vi "Monitors_v01.vi"() -> ()   [LabVIEW 2013]
uses:
  <vilib>/Analysis/5stat.llb/RMS (DBL).vi
  <vilib>/Analysis/baseanly.llb/Mean (DBL).vi
  <vilib>/measure/macond.llb/IIR Filter for N Chan.vi
  Global VIs/shotnoise.vi
  <vilib>/Analysis/NI_AALPro.lvlib
  <vilib>/Analysis/NI_AALBase.lvlib
  <vilib>/measure/NI_MAPro.lvlib
panel:
  in  "IIR filter specifications":T1={"Topology"=enum."Butterworth", "Type"=enum."Lowpass", "Order"=1, "Lower Fc"=100.0, "Upper Fc"=200.0, "PB Ripple"=1.0, "SB Attenuation"=60.0} {"PB Ripple" format="%0.2f"; "SB Attenuation" format="%0.2f"; "Lower Fc" format="%0.2p"; "Upper Fc" format="%0.2p"}
  in  "Shot noise start":bool
  out "Variance 1 normalised to SNL":dbl(graph)
  out "Variance 2 normalised to SNL":dbl(graph)
  out "conditional variance":dbl
  out "covariance":dbl
  out "Signal 2":dbl[](graph)
  out "Signal 1":dbl[](graph)
  in  "wfm":waveform(dbl)[](array[waveform]) caption="波形"
types:
  T1 = cluster{"Topology":enum16{"Off", "Butterworth", "Chebyshev", "Inverse Chebyshev", "Elliptic", "Bessel"}, "Type":enum16{"Lowpass", "Highpass", "Bandpass", "Bandstop"}, "Order":i32, "Lower Fc":dbl, "Upper Fc":dbl, "PB Ripple":dbl, "SB Attenuation":dbl}
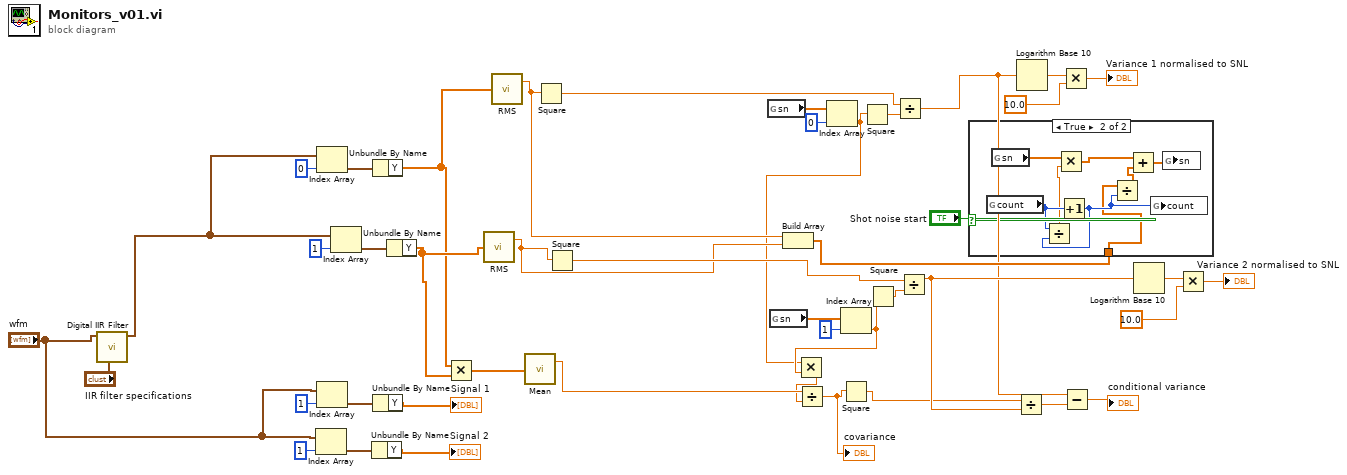
[diagram p0: block diagram]
diagram:
  n1 = call-poly <vilib>:"Digital IIR Filter.vi"("IIR filter specifications"="IIR filter specifications", "signal(s) in"="wfm") -> ("signal(s) out"=w1:waveform(dbl)[])  [unwired: 4 in, 5 out]
  n2 = Index Array(array="wfm", index=1) -> (element=w40:waveform(dbl))
  n3 = Index Array(array=w1, index=0) -> (element=w12:waveform(dbl))
  n4 = Index Array(array="wfm", index=1) -> (element=w43:waveform(dbl))
  n5 = Index Array(array=w1, index=1) -> (element=w17:waveform(dbl))
  n6 = Unbundle By Name(w40) -> ("Y"=→"Signal 2":dbl[])
  n7 = Unbundle By Name(w12) -> ("Y"=w36:dbl[])
  n8 = Unbundle By Name(w43) -> ("Y"=→"Signal 1":dbl[])
  n9 = Unbundle By Name(w17) -> ("Y"=w38:dbl[])
  n10 = Multiply(x=w36, y=w38) -> (x*y=w34:dbl[])
  n11 = call-poly <vilib>:"RMS.vi"("X"=w38) -> ("rms value"=w32:dbl)  [unwired: 1 out]
  n12 = call-poly <vilib>:"RMS.vi"("X"=w36) -> ("rms value"=w30:dbl)  [unwired: 1 out]
  n13 = call-poly <vilib>:"Mean.vi"("X"=w34) -> ("mean"=w35:dbl)  [unwired: 1 out]
  n14 = Square(x=w30) -> (x^2=w31:dbl)
  n15 = Square(x=w32) -> (x^2=w33:dbl)
  n16 = global read "shotnoise.vi" "sn"() -> (w14:dbl[])
  n17 = global read "shotnoise.vi" "sn"() -> (w15:dbl[])
  n18 = Build Array(w30, w32) -> (w29:dbl[])
  n19 = Index Array(array=w14, index=0) -> (element=w25:dbl)
  n20 = Index Array(array=w15, index=1) -> (element=w26:dbl)
  n21 = Multiply(x=w25, y=w26) -> (x*y=w27:dbl)
  n22 = Divide(x=w35, y=w27) -> (x/y=w37:dbl)
  "covariance" <- w37
  n23 = Square(x=w37) -> (x^2=w19:dbl)
  n24 = Square(x=w25) -> (x^2=w22:dbl)
  n25 = Square(x=w26) -> (x^2=w24:dbl)
  n26 = Divide(x=w31, y=w22) -> (x/y=w23:dbl)
  n27 = Divide(x=w33, y=w24) -> (x/y=w28:dbl)
  n28 = case shown="True" "Shot noise start" {
    tunnel: w29 -> [_ w46]
    frame False {
    }
    frame True {
      n29 = global read "shotnoise.vi" "count"() -> (w51:i64)
      n30 = global read "shotnoise.vi" "sn"() -> (w50:dbl[])
      n31 = Increment(x=w51) -> (x+1=w47:i64)
      n32 = Divide(x=w51, y=w47) -> (x/y=w49:dbl)
      n33 = Multiply(x=w50, y=w49) -> (x*y=w48:dbl[])
      n34 = Divide(x=w46, y=w47) -> (x/y=w45:dbl[])
      n35 = Add(x=w48, y=w45) -> (x+y=w52:dbl[])
      n36 = global write "shotnoise.vi" "count"(w47) -> ()
      n37 = global write "shotnoise.vi" "sn"(w52) -> ()
    }
  }
  n38 = Divide(x=w19, y=w28) -> (x/y=w20:dbl)
  n39 = Logarithm Base 10(1:w23) -> (0:w4:dbl)
  n40 = Multiply(x=w4, y=10.0) -> (x*y=→"Variance 1 normalised to SNL":dbl)
  n41 = Subtract(x=w23, y=w20) -> (x-y=→"conditional variance":dbl)
  n42 = Logarithm Base 10(1:w28) -> (0:w7:dbl)
  n43 = Multiply(x=w7, y=10.0) -> (x*y=→"Variance 2 normalised to SNL":dbl)
